vi "Write QueueName.vi"(8 "error in (no error)":errorcluster, 10 "QueueName":string, 11 "AWS_SQS in":refnum<class "AWS_SQS.lvclass">) -> (0 "error out":errorcluster, 3 "AWS_SQS out":refnum<class "AWS_SQS.lvclass">)   [LabVIEW 2015, in "AWS_SQS.lvlib" / "AWS_SQS.lvclass"]
uses:
  AWS_SQS.lvclass
  AWS_SQS.lvclass/AWS_SQS.ctl
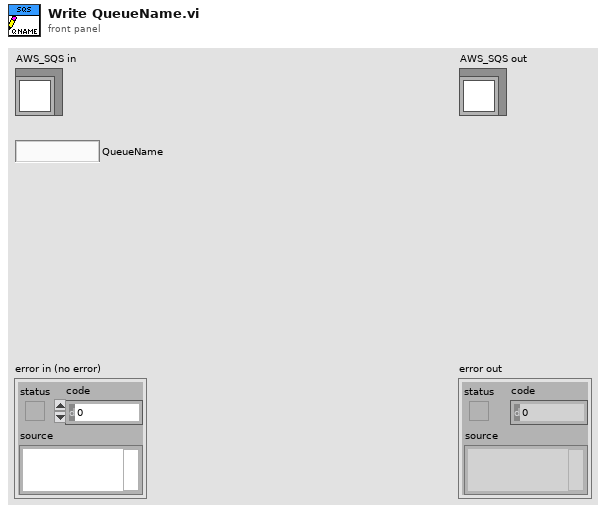
[diagram p1: front panel]
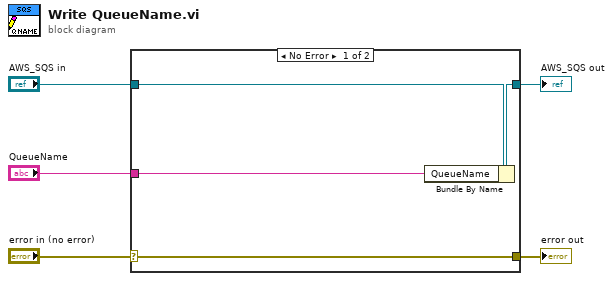
[diagram p0: block diagram]
diagram:
  n1 = case shown="No Error" "error in (no error)" {
    selector: "error in (no error)" -> [w9 w10]
    tunnel: [w9 w10] -> w4
    tunnel: [w7 w11] -> w2
    tunnel: "AWS_SQS in" -> [w8 w11]
    tunnel: "QueueName" -> [w6 _]
    frame No Error {
      n2 = Bundle By Name(cluster=w8, "QueueName"=w6) -> (w7:refnum<class "AWS_SQS.lvclass">)
    }
    frame Error {
    }
  }
  "error out" <- w4
  "AWS_SQS out" <- w2
